vi "Init.vi"() -> (2 "Transport":refnum<class "Transport.lvclass">)   [LabVIEW 2025, in "jettl.lvlib" / "Transport.lvlib" / "Queue.lvlib"]
uses:
  Queue.lvlib
  Transport/Transport.lvclass
  Queue Transport/Queue Transport.lvclass
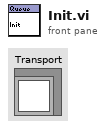
[diagram p1: front panel]
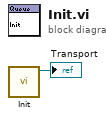
[diagram p0: block diagram]
diagram:
  n1 = call "Init.vi"() -> ("Queue Transport out"=→"Transport":refnum<class "Queue Transport.lvclass">)  [unwired: 11 in]
